vi "Create Custom Device.vi"(8 "error in (no error)":errorcluster, 9 "J1939 Monitor Settings":T2 {"Name" format="%.0x"}, 10 "J1939 XNET Settings":T3={"XNET Database"="", "XNET Cluster"="", "CAN Port"="", "Baud rate [Bd]"=0, "Termination"=0, "Incoming Rate"=0, "Outcoming Rate"=0, "Write Decimation"=100} {"Termination" items=["Off", "On"]}, 11 "Name":string) -> (0 "error out":errorcluster, 2 "Monitor Ref out":T1 format="%.0x", 3 "Custom Device reference":refnum<k24>)   [LabVIEW 2015, in "J1939 System Definition API.lvlib"]
uses:
  J1939 System Definition API.lvlib
  NationalInstruments.VeriStand.SystemDefinitionAPI
  Shared/Types/XNET Settings.ctl
  Shared/Types/Monitor Settings.ctl
  <vilib>/NI Veristand/Custom Device API/Custom Device Item Ref.ctl
  Shared/SubVIs/Constants.vi
  <vilib>/NI Veristand/Custom Device API/Set Item Property (Variant).vi
  Shared/J1939 Addon Shared.lvlib
  <vilib>/NI VeriStand/Custom Device API/Custom Device API.lvlib
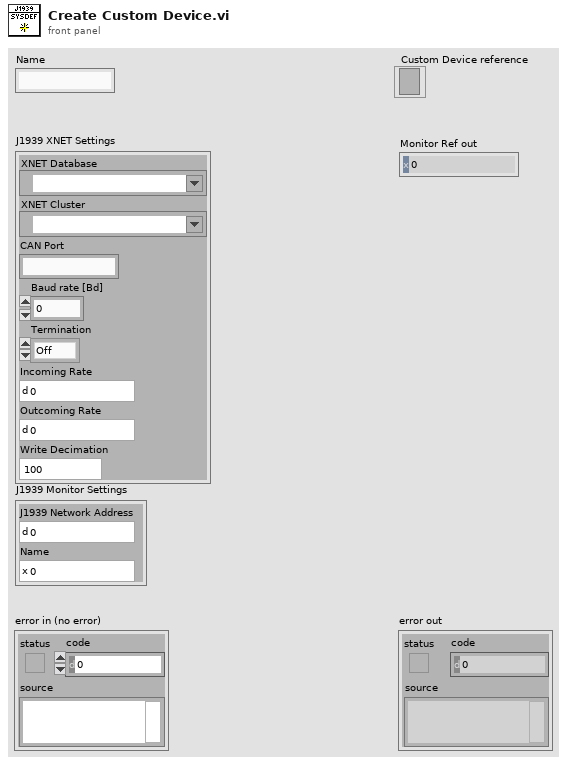
[diagram p1: front panel]
types:
  T1 = typedef "Custom Device API.lvlib/Custom Device Item Ref.ctl" = u64
  T2 = typedef "J1939 Addon Shared.lvlib/Monitor Settings.ctl" = cluster{"J1939 Network Address":u8, "Name":u64}
  T3 = typedef "J1939 Addon Shared.lvlib/XNET Settings.ctl" = cluster{"XNET Database":refnum<k21>, "XNET Cluster":refnum<k21>, "CAN Port":string, "Baud rate [Bd]":u32, "Termination":u32, "Incoming Rate":u32, "Outcoming Rate":u32, "Write Decimation":u32}
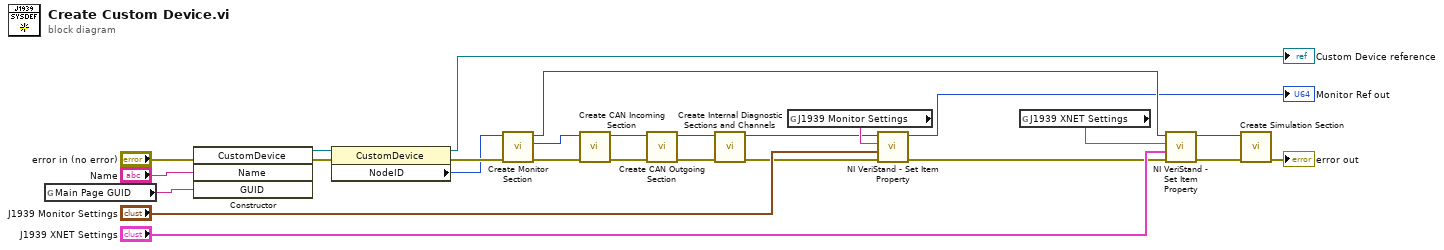
[diagram p0: block diagram]
diagram:
  n1 = global read "Constants.vi" "Main Page GUID"() -> (w21:string)
  n2 = constructor class="CustomDevice"(error in="error in (no error)", "Name"="Name", "GUID"=w21) -> (reference out=w24:refnum<k24>, error out=w23:errorcluster)  [unwired: 2 in, 3 out]
  n3 = property class="CustomDevice"(reference=w24, error in=w23) -> (reference out=→"Custom Device reference":refnum<k24>, error out=w14:errorcluster, "NodeID"=w12:u64)
  n4 = call "Create Monitor Section.vi"("error in (no error)"=w14, "Device Item Ref in"=w12) -> ("error out"=w13:errorcluster, "Section Ptr"=w11:T1, "Parent Ref out"=w8:T1)  [unwired: 7 in]
  n5 = call "Create CAN Incoming Section.vi"("error in (no error)"=w13, "Device Item Ref in"=w11) -> ("error out"=w17:errorcluster, "Device Item Ref Out"=w18:T1)  [unwired: 8 in]
  n6 = call "Create CAN Outgoing Section.vi"("error in (no error)"=w17, "Parent Ref in"=w18) -> ("error out"=w20:errorcluster, "Parent Ref out"=w19:T1)  [unwired: 8 in]
  n7 = call "Create Internal Diagnostic Sections and Channels.vi"("error in (no error)"=w20, "Device Item Ref in"=w19) -> ("error out"=w4:errorcluster, "Device Item Ref Out"=w2:T1)  [unwired: 8 in]
  n8 = global read "Constants.vi" "J1939 Monitor Settings"() -> (w6:string)
  n9 = call-poly <vilib>:"NI VeriStand - Set Item Property.vi"("error in (no error)"=w4, "Value"="J1939 Monitor Settings", "Property Name"=w6, "Item Ref in"=w2) -> ("error out"=w3:errorcluster, "Item Ref out"=→"Monitor Ref out":T1)  [unwired: 5 in, 1 out]
  n10 = global read "Constants.vi" "J1939 XNET Settings"() -> (w16:string)
  n11 = call-poly <vilib>:"NI VeriStand - Set Item Property.vi"("error in (no error)"=w3, "Value"="J1939 XNET Settings", "Property Name"=w16, "Item Ref in"=w8) -> ("error out"=w10:errorcluster, "Item Ref out"=w7:T1)  [unwired: 5 in, 1 out]
  n12 = call "Create Simulation Section.vi"("error in (no error)"=w10, "Parent Ref in"=w7) -> ("error out"=→"error out":errorcluster)  [unwired: 7 in, 2 out]
